vi "create c Daq.vi"(0 "device":string, 1 "digital_io_id":i32[](array[numeric])=[0, 0, 0, 0, 0, 0, 0, 0, 0, 0, 0, 0, 0, 0, 0, 0, 0, 0, 0, 0, 0, 0, 0, 0, 0, 0, 0, 0, 0, 0, 0, 0], 2 "analog_co_io_id":i32[](array[numeric])=[0, 0, 0, 0, 0, 0, 0, 0, 0, 0, 0, 0, 0, 0, 0, 0, 0, 0, 0, 0, 0, 0, 0, 0, 0, 0, 0, 0, 0, 0, 0, 0], 3 "digital_co_io_id":i32[](array[numeric])=[0, 0, 0, 0, 0, 0, 0, 0, 0, 0, 0, 0, 0, 0, 0, 0, 0, 0, 0, 0, 0, 0, 0, 0, 0, 0, 0, 0, 0, 0, 0, 0], 5 "analog_count":i32, 7 "analog_io_id":i32[](array[numeric])=[0, 0, 0, 0, 0, 0, 0, 0, 0, 0, 0, 0, 0, 0, 0, 0, 0, 0, 0, 0, 0, 0, 0, 0, 0, 0, 0, 0, 0, 0, 0, 0], 9 "digital_count":i32, 12 "analog_co_count":i32, 13 "digital_co_count":i32) -> (4 "digital_io_id out":i32[](array[numeric]), 6 "analog_co_io_id out":i32[](array[numeric]), 8 "analog_io_id out":i32[](array[numeric]), 10 "digital_co_io_id out":i32[](array[numeric]), 14 "function return":u32)   [LabVIEW 2020, in "cDaq.lvlib"]
doc: "DAQAPI HDAQ create_cDaq(const char* device,\n const int analog_count, int analog_io_id[32],\n const int digital_count, int digital_io_id[32],\n const int analog_co_count, int analog_co_io_id[32],\n const int digital_co_count, int digital_co_io_id[32]);"
uses:
  cDaq.lvlib
  <userlib>/cDaq/cDaq.dll
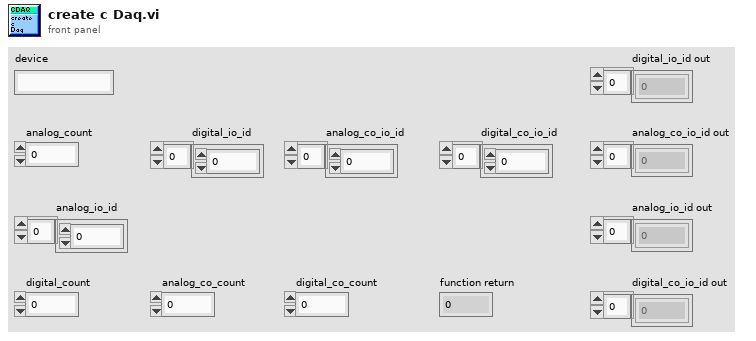
[diagram p1: front panel]
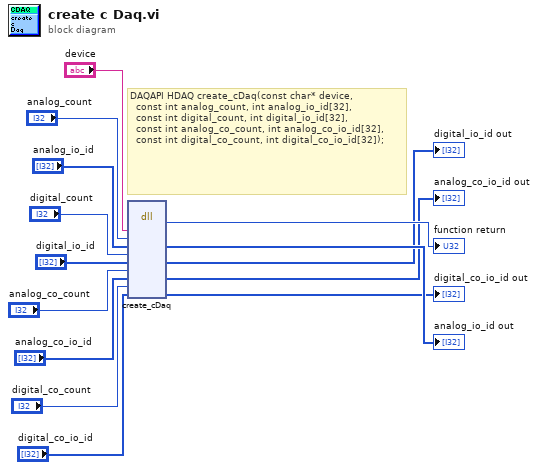
[diagram p0: block diagram]
diagram:
  # "DAQAPI HDAQ create_cDaq(const char* device,\n\t\tconst int analog_count, int analog_io_id[32],\n\t\tconst int digital_count, int digital_io_id[32],\n\t\tconst int analog_co_count, int analog_co_io_id[32],\n\t\tconst int digital_co_count, int digital_co_io_id[32]);"
  n1 = dll-call lib="C:/Program Files (x86)/National Instruments/LabVIEW 2020/user.lib/cDaq/cDaq.*" fn="create_cDaq"("device"="device", "analog_count"="analog_count", "analog_io_id"="analog_io_id", "digital_count"="digital_count", "digital_io_id"="digital_io_id", "analog_co_count"="analog_co_count", "analog_co_io_id"="analog_co_io_id", "digital_co_count"="digital_co_count", "digital_co_io_id"="digital_co_io_id") -> ("type de retour"=→"function return":u32, "analog_io_id"=→"analog_io_id out":i32[], "digital_io_id"=→"digital_io_id out":i32[], "analog_co_io_id"=→"analog_co_io_id out":i32[], "digital_co_io_id"=→"digital_co_io_id out":i32[])  [unwired: 8 in, 2 out]
